vi "SetParentInterfaces.vi"(8 "error in":errorcluster, 10 "Parent Interfaces(ClassRef/Path)":variant[](array[variant]), 11 "Class/InterfaceRefIn":refnum<vi>) -> (0 "error out":errorcluster, 3 "Class/InterfaceRefOut":refnum<vi>)   [LabVIEW 2020, in "InterfaceLibrary.lvlib"]
uses:
  InterfaceLibrary.lvlib
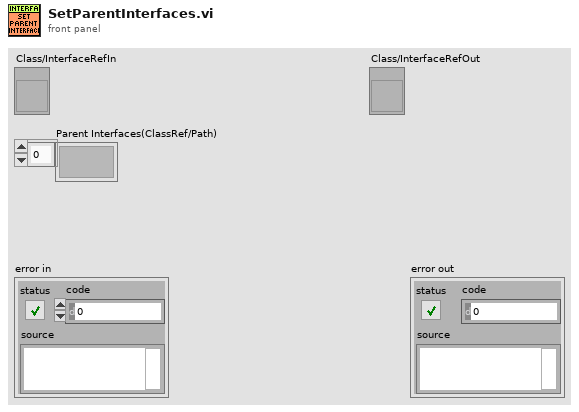
[diagram p1: front panel]
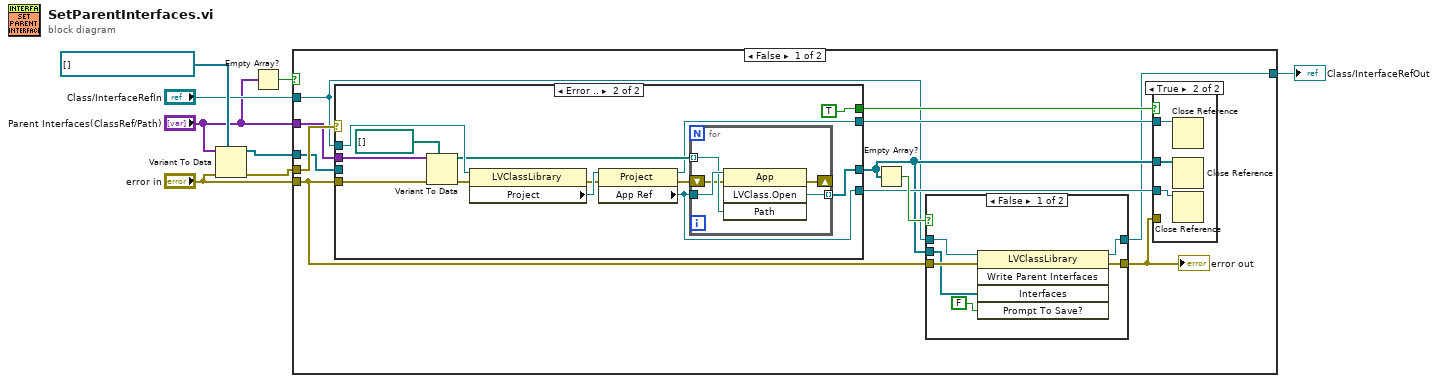
[diagram p0: block diagram]
diagram:
  n1 = Variant To Data(error in="error in", type=refnum<vi>[] [] ("Interface"), Variant="Parent Interfaces(ClassRef/Path)") -> (data=w3:refnum<vi>[], error out=w7:errorcluster)
  n2 = Empty Array?(array="Parent Interfaces(ClassRef/Path)") -> (empty?=w2:bool)
  n3 = case shown="False" w2 {
    tunnel: w7 -> [w19 _]
    tunnel: "Parent Interfaces(ClassRef/Path)" -> [w18 _]
    tunnel: "error in" -> [w13 _]
    tunnel: "Class/InterfaceRefIn" -> [w12 w51]
    tunnel: [w10 w51] -> w4
    tunnel: w3 -> [w9 _]
    frame False {
      n4 = case shown="Error .." w19 {
        tunnel: [w24 w28] -> w14
        tunnel: w9 -> [w24 _]
        tunnel: w18 -> [_ w36]
        tunnel: w12 -> [_ w35]
        tunnel: w13 -> [_ w29]
        tunnel: [_ w27] -> w17
        tunnel: [_ w26] -> w16
        tunnel: [_ TRUE] -> w15
        frame No Error {
        }
        frame Error {
          n5 = Variant To Data(error in=w29, type=path[] [] ("Interface"), Variant=w36) -> (data=w33:path[], error out=w30:errorcluster)
          n6 = property class="LVClassLibrary"(reference=w35, error in=w30) -> (error out=w31:errorcluster, "Project"=w34:refnum<vi>)  [unwired: 1 out]
          n7 = property class="Project"(reference=w34, error in=w31) -> (reference out=w26:refnum<vi>, error out=w32:errorcluster, "App Ref"=w27:refnum<vi>)
          n8 = for {
            tunnel: w27 -> [w42]
            tunnel: w33 -> [w41] mode=indexing
            tunnel: [w39] -> w28 mode=indexing
            shift-right: [w38] -> _
            shift-left: w32 -> [w40]
            n9 = invoke class="App" method="LVClass.Open"(reference=w42, error in=w40, "Path"=w41) -> (error out=w38:errorcluster, "LVClass.Open"=w39:refnum<vi>)  [unwired: 1 in, 2 out]
          }
        }
      }
      n10 = Empty Array?(array=w14) -> (empty?=w20:bool)
      n11 = case shown="False" w20 {
        tunnel: w13 -> [w48 w50]
        tunnel: [w47 w50] -> w11
        tunnel: w12 -> [w46 w49]
        tunnel: [w45 w49] -> w10
        tunnel: w14 -> [w43 _]
        frame False {
          n12 = invoke class="LVClassLibrary" method="Write Parent Interfaces"(reference=w46, error in=w48, "Interfaces"=w43, "Prompt To Save?"=FALSE) -> (reference out=w45:refnum<vi>, error out=w47:errorcluster)  [unwired: 1 in, 3 out]
        }
        frame True {
        }
      }
      "error out" <- w11
      n13 = case shown="True" w15 {
        tunnel: w17 -> [_ w23]
        tunnel: w16 -> [_ w22]
        tunnel: w11 -> [_ _]
        tunnel: w14 -> [_ w21]
        frame False {
        }
        frame True {
          n14 = Close Reference(reference=w22) -> ()  [unwired: 1 in, 1 out]
          n15 = Close Reference(reference=w21) -> ()  [unwired: 1 in, 1 out]
          n16 = Close Reference(reference=w23) -> ()  [unwired: 1 in, 1 out]
        }
      }
    }
    frame True {
    }
  }
  "Class/InterfaceRefOut" <- w4
